vi "Tidal Eng-TCP Example.vi"() -> ()   [LabVIEW 2023]
panel:
  in  "address":string="10.2.0.248"
  in  "remote port or service name":u16=5000
  in  "timeout ms (60000)":i32
  in  "mode (standard)":T1(ring)
  out "data out":string
  in  "bytes to read":i32
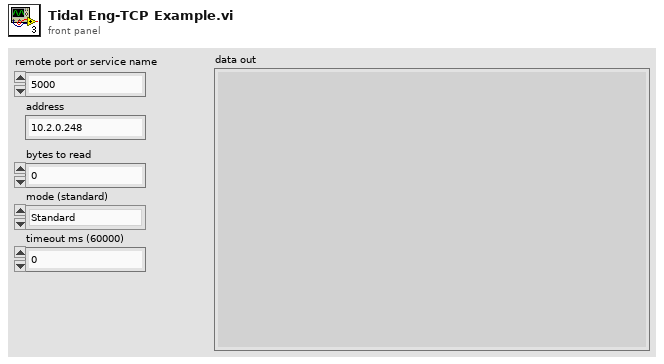
[diagram p1: front panel]
types:
  T1 = enum16{"Standard", "Buffered", "CRLF", "Immediate"}
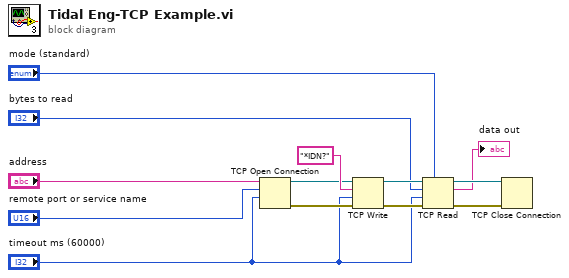
[diagram p0: block diagram]
diagram:
  n1 = TCP Open Connection(address="address", remote port or service name="remote port or service name", timeout ms (60000)="timeout ms (60000)") -> (connection ID=w4:refnum<k5>, error out=w5:errorcluster)  [unwired: 2 in]
  n2 = TCP Write(connection ID=w4, data in="*IDN?" ("ID Query"), error in (no error)=w5, 9:"timeout ms (60000)") -> (connection ID out=w13:refnum<k5>, error out=w11:errorcluster)  [unwired: 1 out]
  n3 = TCP Read(connection ID=w13, bytes to read="bytes to read", error in (no error)=w11, 7:"mode (standard)", 9:"timeout ms (60000)") -> (connection ID out=w12:refnum<k5>, data out=→"data out":string, error out=w10:errorcluster)
  n4 = TCP Close Connection(connection ID=w12, error in (no error)=w10) -> ()  [unwired: 1 in, 2 out]
